vi "GetConfigurationFilePath.vi"() -> (3 "Configuration File Path":path)   [LabVIEW 2019]
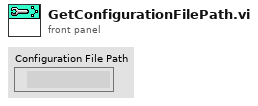
[diagram p1: front panel]
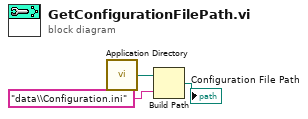
[diagram p0: block diagram]
diagram:
  n1 = call <vilib>:"Application Directory.vi"() -> ("Application Directory"=w1:path)
  n2 = Build Path(base path=w1, name or relative path="data\\Configuration.ini") -> (appended path=→"Configuration File Path":path)
